vi "Supplementary Fig.11b-2.vi"() -> ()   [LabVIEW 2018]
panel:
  in  "file type":string=".info"
  out "files":string[](array[string])
  in  "filepath":path
  out "area":dbl[](array[numeric])
  in  "Cluster":T1={"index"=1, "upper limit"=7.0, "lower limit"=5.6000000000000005, "Boolean"=TRUE}
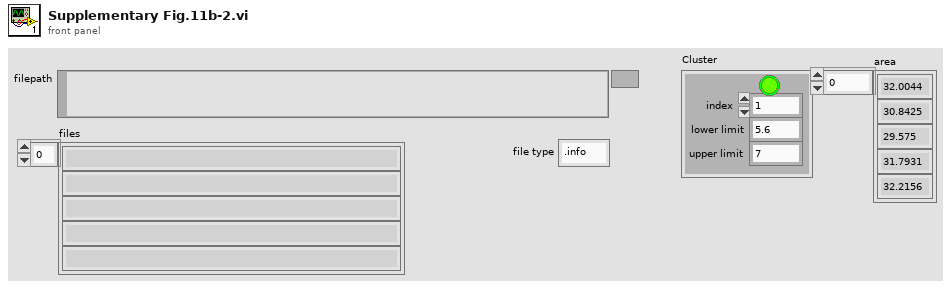
[diagram p1: front panel]
types:
  T1 = cluster{"index":i32, "upper limit":dbl, "lower limit":dbl, "Boolean":bool}
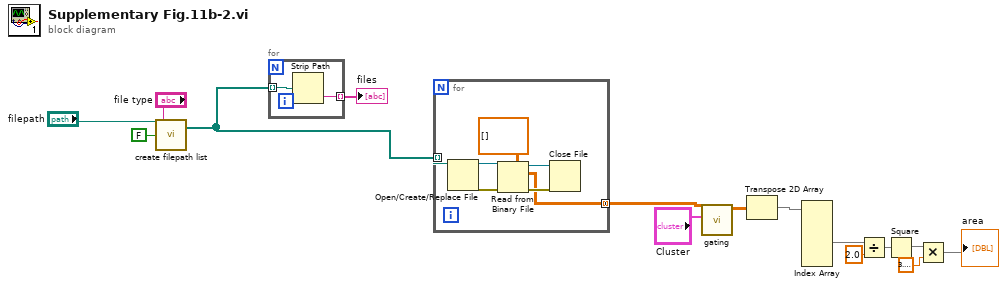
[diagram p0: block diagram]
diagram:
  n1 = call "create filepath list.vi"("regular expression"="file type", "search subholder"=FALSE, "path"="filepath") -> ("Array"=w7:path[])  [unwired: 1 out]
  n2 = for {
    tunnel: w7 -> [w17] mode=indexing
    tunnel: [w16] -> w2 mode=indexing
    n3 = Strip Path(path=w17) -> (name=w16:string)  [unwired: 1 out]
  }
  "files" <- w2
  n4 = for {
    tunnel: [w19] -> w6 mode=concatenating
    tunnel: w7 -> [w18] mode=indexing
    n5 = Open/Create/Replace File(file path (use dialog)=w18) -> (refnum out=w22:refnum<file>, error out=w21:errorcluster)  [unwired: 5 in, 1 out]
    n6 = Read from Binary File(5:dbl[][] [], 8:w21, 11:w22) -> (0:w24:errorcluster, 2:w19:dbl[][], 3:w23:refnum<file>)  [unwired: 3 in, 1 out]
    n7 = Close File(refnum=w23, error in=w24) -> ()  [unwired: 2 out]
  }
  n8 = call "gating.vi"("Cluster"="Cluster", "Array in"=w6) -> ("Array out"=w14:dbl[][])  [unwired: 8 in, 1 out]
  n9 = Transpose 2D Array(2D array=w14) -> (transposed array=w5:dbl[][])
  n10 = Index Array(array=w5) -> (element #2=w9:dbl[])  [unwired: 6 in, 2 out]
  n11 = Divide(x=w9, y=2.0) -> (x/y=w12:dbl[])
  n12 = Square(x=w12) -> (x^2=w13:dbl[])
  n13 = Multiply(x=w13, y=3.141592653589793) -> (x*y=→"area":dbl[])
